vi "Find VI.vi"(10 "Framework VI to Find":T1, 11 "Library in":refnum<vi>) -> (3 "Framework VI Path":path)   [LabVIEW 2019, in "Panther Dashboard.lvlib"]
uses:
  Panther Dashboard.lvlib
  Public VIs names--enum.ctl
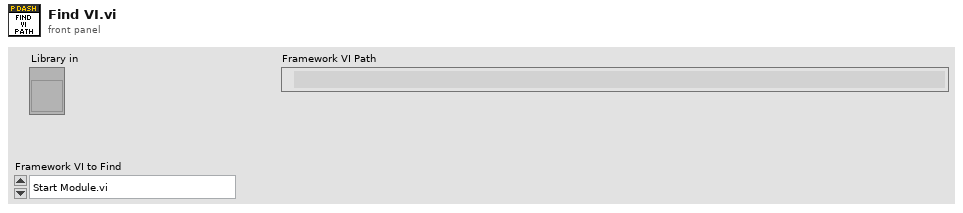
[diagram p1: front panel]
types:
  T1 = typedef "Panther Dashboard.lvlib/Public VIs names--enum.ctl" = enum16{"Start Module.vi", "Synchronize Module Events.vi", "Obtain Broadcast Events for Registration.vi", "Null Broadcast Events--constant.vi", "Stop Module.vi"}
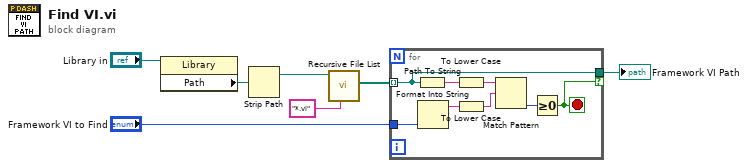
[diagram p0: block diagram]
diagram:
  n1 = property class="Library"(reference="Library in") -> ("Path"=w3:path)  [unwired: 1 in, 2 out]
  n2 = Strip Path(path=w3) -> (stripped path=w2:path)  [unwired: 1 out]
  n3 = call <vilib>:"Recursive File List.vi"("pattern"="*.vi", "Folder Path"=w2) -> ("All Files in Dir"=w5:path[])  [unwired: 5 in, 4 out]
  n4 = for {
    tunnel: "Framework VI to Find" -> [w15]
    tunnel: w5 -> [w11] mode=indexing
    tunnel: [w11] -> w4 if=w10
    stop <- w10 stop-if-true
    n5 = Path To String(path=w11) -> (string=w13:string)
    n6 = Format Into String(w15) -> (resulting string=w14:string)  [unwired: 3 in, 1 out]
    n7 = To Lower Case(string=w13) -> (all lower case string=w9:string)
    n8 = To Lower Case(string=w14) -> (all lower case string=w8:string)
    n9 = Match Pattern(string=w9, regular expression=w8) -> (offset past match=w12:i32)  [unwired: 1 in, 3 out]
    n10 = Greater Or Equal To 0?(x=w12) -> (x >= 0?=w10:bool)
  }
  "Framework VI Path" <- w4
